vi "矩阵转置.vi"() -> ()   [LabVIEW 2018]
uses:
  <vilib>/Analysis/Matrix/Datatypes/RealMatrix.ctl
  <vilib>/Analysis/7linalg.llb/Real Transpose Matrix.vi
  <vilib>/Analysis/NI_AALPro.lvlib
  <vilib>/Analysis/Matrix/NI_Matrix.lvlib
panel:
  out "Matrix Transpose":T1 caption="矩阵转置"
  in  "Real Matrix":T1 caption="实数矩阵"
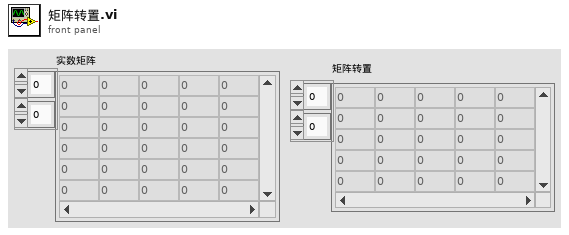
[diagram p1: front panel]
types:
  T1 = typedef "NI_Matrix.lvlib/RealMatrix.ctl" = dbl[][]
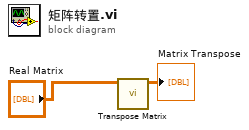
[diagram p0: block diagram]
diagram:
  n1 = call-poly <vilib>:"Transpose Matrix.vi"("Input Matrix"="Real Matrix") -> ("Matrix Transpose"=→"Matrix Transpose":T1)  [unwired: 9 in, 1 out]
